vi "SetListener.vi"(8 "error in (no error)":errorcluster, 10 "Listener":refnum<class "TestListener.lvclass">, 11 "TestResult in":refnum<class "TestResult.lvclass">) -> (0 "error out":errorcluster, 3 "TestResult out":refnum<class "TestResult.lvclass">)   [LabVIEW 2019, in "TestResult.lvclass"]
doc: "Sets the <B>TestListener</B>."
uses:
  TestResult.lvclass
  TestListener/TestListener.lvclass
  TestResult.lvclass/TestResult.ctl
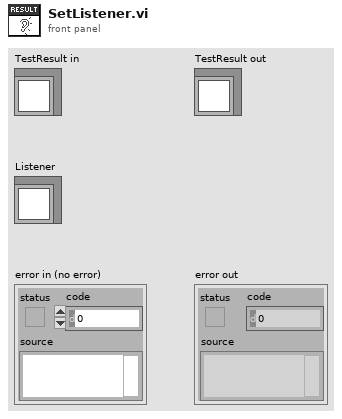
[diagram p1: front panel]
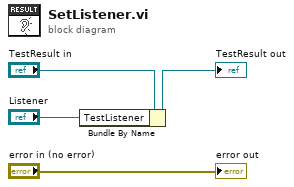
[diagram p0: block diagram]
diagram:
  n1 = Bundle By Name(cluster="TestResult in", "TestListener"="Listener") -> (→"TestResult out":refnum<class "TestResult.lvclass">)
  "error out" <- "error in (no error)"
